vi "commit.vi"(8 "error in (no error)":errorcluster, 11 "lv-builder-default in":refnum<class "lv-builder-default.lvclass">) -> (0 "error out":errorcluster, 3 "lv-builder-default out":refnum<class "lv-builder-default.lvclass">)   [LabVIEW 2015, in "lv-builder-default.lvclass"]
uses:
  lv-builder-default.lvclass
  lv-builder-default.lvclass/lv-builder-default.ctl
  community/_controls/command_configuration.ctl
  community/_controls/version_command.ctl
  lv-builder/public/accessors/project_file_read.vi
  lv-builder-default.lvlib
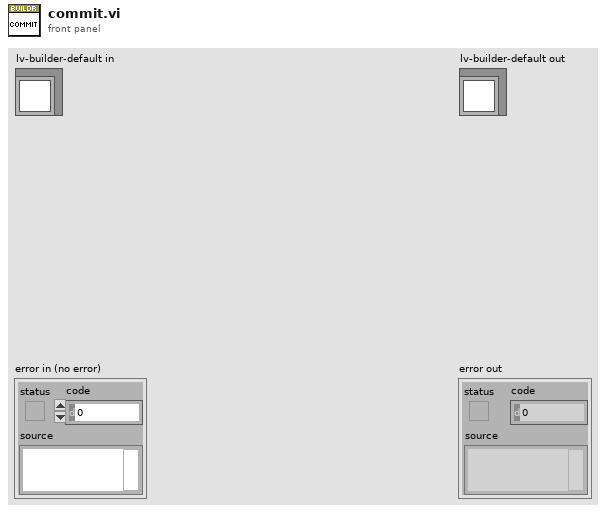
[diagram p1: front panel]
types:
  T1 = typedef "lv-builder-default.lvlib/version_command.ctl" = enum16{"<version_command>", "read_config", "write_config", "<null>"}
  T2 = typedef "lv-builder-default.lvlib/command_configuration.ctl" = enum16{"<config_command>", "read_config", "write_config", "<null>"}
  T3 = typedef "lv-builder-default.lvlib/configuration.ctl" = cluster{"project_file":string, "lvlibp_directory":string, "zip_directory":string, "lvlib_directory":string, "update_version_vi":string, "installer_post_file":string, "distribution_folder":string, "dependencies_folder":string, "bin_folder":string, "lvlib_post_action":u16, "installer_post_action":u16, "application_post_action":u16, "zip_post_action":u16}
  T4 = typedef "lv-builder-default.lvlib/version.ctl" = cluster{"project_file":string, "major":u32, "minor":u32, "fix":u32, "build":u32, "last_built":dbl, "suffix":string, "auto_increment":bool}
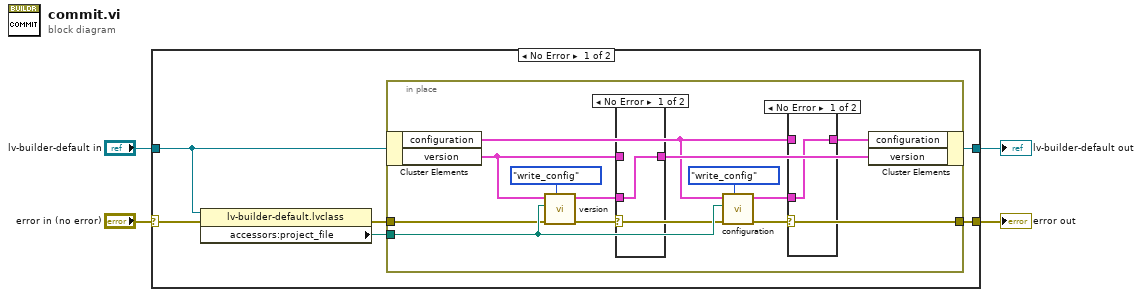
[diagram p0: block diagram]
diagram:
  n1 = case shown="No Error" "error in (no error)" {
    selector: "error in (no error)" -> [w7 w27]
    tunnel: "lv-builder-default in" -> [w8 w28]
    tunnel: [w10 w28] -> w3
    tunnel: [w9 w27] -> w2
    frame No Error {
      n2 = property class="lv-builder-default.lvclass"(reference=w8, error in=w7) -> (error out=w6:errorcluster, "accessors:project_file"=w5:path)  [unwired: 1 out]
      n3 = in-place {
        in-place-border: w6 -> [w14]
        in-place-border: [w18] -> w9
        in-place-border: w5 -> [w15]
        n4 = in-place-cluster #1(w8) -> ("configuration"=w12:T3, "version"=w13:T4)
        n5 = call "version.vi"("command"=version_command."write_config", "error in (no error)"=w14, "project_file"=w15, "version in"=w13) -> ("error out"=w11:errorcluster, "version out"=w16:T4)  [unwired: 6 in]
        n6 = case shown="No Error" w11 {
          tunnel: w13 -> [_ w24]
          tunnel: [w23 w24] -> w20
          tunnel: w16 -> [w23 _]
          frame No Error {
          }
          frame Error {
          }
        }
        n7 = call "configuration.vi"("command"=command_configuration."write_config", "error in (no error)"=w11, "project_file"=w15, "config in"=w12) -> ("error out"=w18:errorcluster, "config out"=w19:T3)  [unwired: 6 in]
        n8 = case shown="No Error" w18 {
          tunnel: w19 -> [w25 _]
          tunnel: w12 -> [_ w26]
          tunnel: [w25 w26] -> w17
          frame No Error {
          }
          frame Error {
          }
        }
        n9 = in-place-cluster #1("configuration"=w17, "version"=w20) -> (w10:refnum<class "lv-builder-default.lvclass">)
      }
    }
    frame Error {
    }
  }
  "error out" <- w2
  "lv-builder-default out" <- w3
